vi "FTW-Endpoint-TCP-Receive-Worker-Start.vi"(0 "FTW-Endpoint-TCP In":refnum<class "FTW-Endpoint-TCP.lvclass">, 5 "Endpoint Address":string, 11 "error in":errorcluster) -> (4 "FTW-Endpoint-TCP Out":refnum<class "FTW-Endpoint-TCP.lvclass">, 15 "error out":errorcluster)   [LabVIEW 2013, in "FTW-Endpoint-TCP.lvclass"]
uses:
  FTW-Endpoint-TCP.lvclass
  FTW-Endpoint-TCP-Receive-Worker.vi
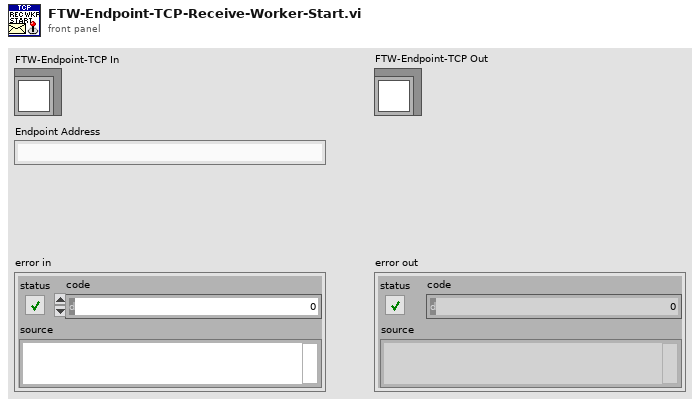
[diagram p1: front panel]
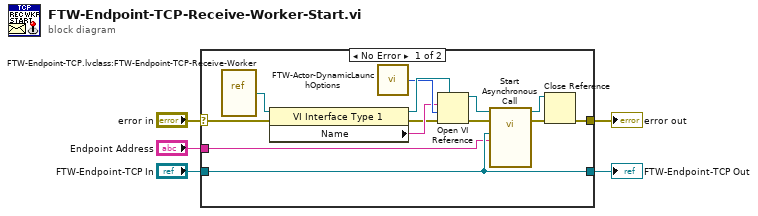
[diagram p0: block diagram]
diagram:
  n1 = case shown="No Error" "error in" {
    selector: "error in" -> [w17 w19]
    tunnel: [w18 w19] -> w1
    tunnel: "Endpoint Address" -> [w6 _]
    tunnel: "FTW-Endpoint-TCP In" -> [w7 w20]
    tunnel: [w7 w20] -> w3
    frame No Error {
      n2 = vi-ref "FTW-Endpoint-TCP.lvclass:FTW-Endpoint-TCP-Receive-Worker.vi"() -> (w8:refnum<vi>)
      n3 = property class="VI Interface Type 1"(reference=w8, error in=w17) -> (reference out=w12:refnum<vi>, error out=w9:errorcluster, "Name"=w10:string)
      n4 = call "FTW-Actor-DynamicLaunchOptions.vi"() -> ("Open VI Ref Options"=w11:i32)
      n5 = Open VI Reference(type specifier VI Refnum (for type only)=w12, vi path=w10, options=w11, error in (no error)=w9) -> (vi reference=w14:refnum<vi>, error out=w16:errorcluster)  [unwired: 2 in]
      n6 = call-by-ref "Start Asynchronous Call"(reference=w14, error in=w16, "TCP Endpoint"=w7, "Address"=w6) -> (reference out=w15:refnum<vi>, error out=w13:errorcluster)  [unwired: 14 in]
      n7 = Close Reference(reference=w15, error in (no error)=w13) -> (error out=w18:errorcluster)
    }
    frame Error {
    }
  }
  "FTW-Endpoint-TCP Out" <- w3
  "error out" <- w1
